vi "(SubVI)DW7912.vi"() -> ()   [LabVIEW 2020]
uses:
  Controls/(Ctrl)DW7912_Wave Seq.ctl
  System Command/Controls/(Ctrl)System Command_Trig GPIO Control.ctl
  <vilib>/Utility/miscctls.llb/LVPointTypeDef.ctl
  Control Data/Controls/(Ctrl)Control Data_Save or Load Control Data_Function.ctl
  Libraries/Haptic IC Class/Haptic IC/Haptic IC.lvclass/Haptic IC.ctl
  I2C/Controls/(Ctrl)I2C_8Bit_Read Array.ctl
  Waveform Editor/Controls/(Ctrl)Waveform Editor_Update Sampling Rate Value.ctl
  a7fdcbe2-e318-4fc3-ac41-e38a3fe8abb3.vi
  Libraries/Haptic IC Class/Haptic IC/Accessors/Write freq ref.vi
  Libraries/Haptic IC Class/Haptic IC/Accessors/Write voltage range ref.vi
  Libraries/Haptic IC Class/Haptic IC/Accessors/Write mode ref.vi
  Variables/(Var)System Variables.vi
  I2C/Instance VIs/(SubVI)I2C_8Bit-8Bit_Read_Single.vi
  I2C/Instance VIs/(SubVI)I2C_8Bit-8Bit_Read_Array.vi
  I2C/Instance VIs/(SubVI)I2C_8Bit-8Bit_Read_Sequential.vi
  I2C/Instance VIs/(SubVI)I2C_8Bit-8Bit_Write_Single.vi
  <vilib>/Comparison/Equal/Equal Functor/Equal Functor.lvclass
  Libraries/Haptic IC Class/Haptic IC/Haptic IC.lvclass
panel:
  in  "Stop":bool
  in  "Read All":bool
  in  "Mode Tab":enum32{"Memory Mode", "Trig Mode"}(tab)
  in  "Mem_Stop":bool
  in  "Mem_Start":bool
  in  "Mem Set_Main Seq Loop":u8(ring) caption="Sequence Loop" items=["X1", "X2", "X3", "X4", "X5", "X6", "X7", "X8", "X9", "X10", "X11", "X12", "X13", "X14", "X15", "Infinite"]
  in  "Mem Set_Gain":u8(ring) caption="MEM Gain" items=["100%", "75%", "50%", "25%"]
  in  "Mem Set_Wave Seq Loop":T1 {"Loop 7" items=["X1", "X2", "X3", "X4", "X5", "X6", "X7", "X8", "X9", "X10", "X11", "X12", "X13", "X14", "X15", "Infinite"]; "Loop 6" items=["X1", "X2", "X3", "X4", "X5", "X6", "X7", "X8", "X9", "X10", "X11", "X12", "X13", "X14", "X15", "Infinite"]; "Loop 5" items=["X1", "X2", "X3", "X4", "X5", "X6", "X7", "X8", "X9", "X10", "X11", "X12", "X13", "X14", "X15", "Infinite"]; "Loop 4" items=["X1", "X2", "X3", "X4", "X5", "X6", "X7", "X8", "X9", "X10", "X11", "X12", "X13", "X14", "X15", "Infinite"]; "Loop 3" items=["X1", "X2", "X3", "X4", "X5", "X6", "X7", "X8", "X9", "X10", "X11", "X12", "X13", "X14", "X15", "Infinite"]; "Loop 2" items=["X1", "X2", "X3", "X4", "X5", "X6", "X7", "X8", "X9", "X10", "X11", "X12", "X13", "X14", "X15", "Infinite"]; "Loop 1" items=["X1", "X2", "X3", "X4", "X5", "X6", "X7", "X8", "X9", "X10", "X11", "X12", "X13", "X14", "X15", "Infinite"]; "Loop 0" items=["X1", "X2", "X3", "X4", "X5", "X6", "X7", "X8", "X9", "X10", "X11", "X12", "X13", "X14", "X15", "Infinite"]}
  in  "Mem Set_Read":bool caption="Wave Sequence"
  in  "Mem Set_Wave Seq":T3 caption="WAVE SEQUENCE" {"Wave Seq. 7"."Seq/Delay" items=["Empty", "1", "2", "3", "4", "5", "6", "7", "8", "9", "10", "11", "12", "13", "14", "15", "16", "17", "18", "19", "20", "21", "22", "23", "24", "25", "26", "27", "28", "29", "30", "31", "32", "33", "34", "35", "36", "37", "38", "39", "40", "41", "42", "43", "44", "45", "46", "47", "48", "49", "50", "51", "52", "53", "54", "55", "56", "57", "58", "59", "60", "61", "62", "63", "64", "65", "66", "67", "68", "69", "70", "71", "72", "73", "74", "75", "76", "77", "78", "79", "80", "81", "82", "83", "84", "85", "86", "87", "88", "89", "90", "91", "92", "93", "94", "95", "96", "97", "98", "99", "100", "101", "102", "103", "104", "105", "106", "107", "108", "109", "110", "111", "112", "113", "114", "115", "116", "117", "118", "119", "120", "121", "122", "123", "124", "125", "126", "127"]; "Wave Seq. 7"."Mode" items=["Wave Seq. 7", "Delay"]; "Wave Seq. 6"."Seq/Delay" items=["Empty", "1", "2", "3", "4", "5", "6", "7", "8", "9", "10", "11", "12", "13", "14", "15", "16", "17", "18", "19", "20", "21", "22", "23", "24", "25", "26", "27", "28", "29", "30", "31", "32", "33", "34", "35", "36", "37", "38", "39", "40", "41", "42", "43", "44", "45", "46", "47", "48", "49", "50", "51", "52", "53", "54", "55", "56", "57", "58", "59", "60", "61", "62", "63", "64", "65", "66", "67", "68", "69", "70", "71", "72", "73", "74", "75", "76", "77", "78", "79", "80", "81", "82", "83", "84", "85", "86", "87", "88", "89", "90", "91", "92", "93", "94", "95", "96", "97", "98", "99", "100", "101", "102", "103", "104", "105", "106", "107", "108", "109", "110", "111", "112", "113", "114", "115", "116", "117", "118", "119", "120", "121", "122", "123", "124", "125", "126", "127"]; "Wave Seq. 6"."Mode" items=["Wave Seq. 6", "Delay"]; "Wave Seq. 5"."Seq/Delay" items=["Empty", "1", "2", "3", "4", "5", "6", "7", "8", "9", "10", "11", "12", "13", "14", "15", "16", "17", "18", "19", "20", "21", "22", "23", "24", "25", "26", "27", "28", "29", "30", "31", "32", "33", "34", "35", "36", "37", "38", "39", "40", "41", "42", "43", "44", "45", "46", "47", "48", "49", "50", "51", "52", "53", "54", "55", "56", "57", "58", "59", "60", "61", "62", "63", "64", "65", "66", "67", "68", "69", "70", "71", "72", "73", "74", "75", "76", "77", "78", "79", "80", "81", "82", "83", "84", "85", "86", "87", "88", "89", "90", "91", "92", "93", "94", "95", "96", "97", "98", "99", "100", "101", "102", "103", "104", "105", "106", "107", "108", "109", "110", "111", "112", "113", "114", "115", "116", "117", "118", "119", "120", "121", "122", "123", "124", "125", "126", "127"]; "Wave Seq. 5"."Mode" items=["Wave Seq. 5", "Delay"]; "Wave Seq. 4"."Seq/Delay" items=["Empty", "1", "2", "3", "4", "5", "6", "7", "8", "9", "10", "11", "12", "13", "14", "15", "16", "17", "18", "19", "20", "21", "22", "23", "24", "25", "26", "27", "28", "29", "30", "31", "32", "33", "34", "35", "36", "37", "38", "39", "40", "41", "42", "43", "44", "45", "46", "47", "48", "49", "50", "51", "52", "53", "54", "55", "56", "57", "58", "59", "60", "61", "62", "63", "64", "65", "66", "67", "68", "69", "70", "71", "72", "73", "74", "75", "76", "77", "78", "79", "80", "81", "82", "83", "84", "85", "86", "87", "88", "89", "90", "91", "92", "93", "94", "95", "96", "97", "98", "99", "100", "101", "102", "103", "104", "105", "106", "107", "108", "109", "110", "111", "112", "113", "114", "115", "116", "117", "118", "119", "120", "121", "122", "123", "124", "125", "126", "127"]; "Wave Seq. 4"."Mode" items=["Wave Seq. 4", "Delay"]; "Wave Seq. 3"."Seq/Delay" items=["Empty", "1", "2", "3", "4", "5", "6", "7", "8", "9", "10", "11", "12", "13", "14", "15", "16", "17", "18", "19", "20", "21", "22", "23", "24", "25", "26", "27", "28", "29", "30", "31", "32", "33", "34", "35", "36", "37", "38", "39", "40", "41", "42", "43", "44", "45", "46", "47", "48", "49", "50", "51", "52", "53", "54", "55", "56", "57", "58", "59", "60", "61", "62", "63", "64", "65", "66", "67", "68", "69", "70", "71", "72", "73", "74", "75", "76", "77", "78", "79", "80", "81", "82", "83", "84", "85", "86", "87", "88", "89", "90", "91", "92", "93", "94", "95", "96", "97", "98", "99", "100", "101", "102", "103", "104", "105", "106", "107", "108", "109", "110", "111", "112", "113", "114", "115", "116", "117", "118", "119", "120", "121", "122", "123", "124", "125", "126", "127"]; "Wave Seq. 3"."Mode" items=["Wave Seq. 3", "Delay"]; "Wave Seq. 2"."Seq/Delay" items=["Empty", "1", "2", "3", "4", "5", "6", "7", "8", "9", "10", "11", "12", "13", "14", "15", "16", "17", "18", "19", "20", "21", "22", "23", "24", "25", "26", "27", "28", "29", "30", "31", "32", "33", "34", "35", "36", "37", "38", "39", "40", "41", "42", "43", "44", "45", "46", "47", "48", "49", "50", "51", "52", "53", "54", "55", "56", "57", "58", "59", "60", "61", "62", "63", "64", "65", "66", "67", "68", "69", "70", "71", "72", "73", "74", "75", "76", "77", "78", "79", "80", "81", "82", "83", "84", "85", "86", "87", "88", "89", "90", "91", "92", "93", "94", "95", "96", "97", "98", "99", "100", "101", "102", "103", "104", "105", "106", "107", "108", "109", "110", "111", "112", "113", "114", "115", "116", "117", "118", "119", "120", "121", "122", "123", "124", "125", "126", "127"]; "Wave Seq. 2"."Mode" items=["Wave Seq. 2", "Delay"]; "Wave Seq. 1"."Seq/Delay" items=["Empty", "1", "2", "3", "4", "5", "6", "7", "8", "9", "10", "11", "12", "13", "14", "15", "16", "17", "18", "19", "20", "21", "22", "23", "24", "25", "26", "27", "28", "29", "30", "31", "32", "33", "34", "35", "36", "37", "38", "39", "40", "41", "42", "43", "44", "45", "46", "47", "48", "49", "50", "51", "52", "53", "54", "55", "56", "57", "58", "59", "60", "61", "62", "63", "64", "65", "66", "67", "68", "69", "70", "71", "72", "73", "74", "75", "76", "77", "78", "79", "80", "81", "82", "83", "84", "85", "86", "87", "88", "89", "90", "91", "92", "93", "94", "95", "96", "97", "98", "99", "100", "101", "102", "103", "104", "105", "106", "107", "108", "109", "110", "111", "112", "113", "114", "115", "116", "117", "118", "119", "120", "121", "122", "123", "124", "125", "126", "127"]; "Wave Seq. 1"."Mode" items=["Wave Seq. 1", "Delay"]; "Wave Seq. 0"."Seq/Delay" items=["Empty", "1", "2", "3", "4", "5", "6", "7", "8", "9", "10", "11", "12", "13", "14", "15", "16", "17", "18", "19", "20", "21", "22", "23", "24", "25", "26", "27", "28", "29", "30", "31", "32", "33", "34", "35", "36", "37", "38", "39", "40", "41", "42", "43", "44", "45", "46", "47", "48", "49", "50", "51", "52", "53", "54", "55", "56", "57", "58", "59", "60", "61", "62", "63", "64", "65", "66", "67", "68", "69", "70", "71", "72", "73", "74", "75", "76", "77", "78", "79", "80", "81", "82", "83", "84", "85", "86", "87", "88", "89", "90", "91", "92", "93", "94", "95", "96", "97", "98", "99", "100", "101", "102", "103", "104", "105", "106", "107", "108", "109", "110", "111", "112", "113", "114", "115", "116", "117", "118", "119", "120", "121", "122", "123", "124", "125", "126", "127"]; "Wave Seq. 0"."Mode" items=["Wave Seq. 0", "Delay"]}
  out "Trig_Gen_Pict":picture
  in  "Trig_Read":bool caption="Trig/Interrupt Mode Set"
  in  "Trig_Gen_Set":bool
  in  "Trig_Mode":bool
  in  "Trig_F Wave":u8(ring) caption="TRIG F Wave" items=["Empty", "1", "2", "3", "4", "5", "6", "7", "8", "9", "10", "11", "12", "13", "14", "15", "16", "17", "18", "19", "20", "21", "22", "23", "24", "25", "26", "27", "28", "29", "30", "31", "32", "33", "34", "35", "36", "37", "38", "39", "40", "41", "42", "43", "44", "45", "46", "47", "48", "49", "50", "51", "52", "53", "54", "55", "56", "57", "58", "59", "60", "61", "62", "63", "64", "65", "66", "67", "68", "69", "70", "71", "72", "73", "74", "75", "76", "77", "78", "79", "80", "81", "82", "83", "84", "85", "86", "87", "88", "89", "90", "91", "92", "93", "94", "95", "96", "97", "98", "99", "100", "101", "102", "103", "104", "105", "106", "107", "108", "109", "110", "111", "112", "113", "114", "115", "116", "117", "118", "119", "120", "121", "122", "123", "124", "125", "126", "127"]
  in  "Trig_R Wave":u8(ring) caption="TRIG R Wave" items=["Empty", "1", "2", "3", "4", "5", "6", "7", "8", "9", "10", "11", "12", "13", "14", "15", "16", "17", "18", "19", "20", "21", "22", "23", "24", "25", "26", "27", "28", "29", "30", "31", "32", "33", "34", "35", "36", "37", "38", "39", "40", "41", "42", "43", "44", "45", "46", "47", "48", "49", "50", "51", "52", "53", "54", "55", "56", "57", "58", "59", "60", "61", "62", "63", "64", "65", "66", "67", "68", "69", "70", "71", "72", "73", "74", "75", "76", "77", "78", "79", "80", "81", "82", "83", "84", "85", "86", "87", "88", "89", "90", "91", "92", "93", "94", "95", "96", "97", "98", "99", "100", "101", "102", "103", "104", "105", "106", "107", "108", "109", "110", "111", "112", "113", "114", "115", "116", "117", "118", "119", "120", "121", "122", "123", "124", "125", "126", "127"]
  in  "Trig_Gen_Setting":T4={"1st Trig"={"Trigger"=TRUE, "Low"=0, "High"=100}, "2nd Trig"={"Trigger"=TRUE, "Low"=0, "High"=100}, "3rd Trig"={"Trigger"=FALSE, "Low"=0, "High"=1}, "4th Trig"={"Trigger"=FALSE, "Low"=0, "High"=1}} {"4th Trig"."High" min=1 max=8000; "4th Trig"."Low" max=7999; "3rd Trig"."High" min=1 max=8000; "3rd Trig"."Low" max=7999; "2nd Trig"."High" min=1 max=8000; "2nd Trig"."Low" max=7999; "1st Trig"."High" min=1 max=8000; "1st Trig"."Low" max=7999}
  in  "Common Tab":enum32{"Common"}(tab)
  in  "Com_Status_Read":bool
  in  "Com_Read":bool caption="Common"
  in  "Com_Bst_VD Clamp":u8(ring) caption="VD Clamp" items=["0.00V", "0.04V", "0.08V", "0.12V", "0.16V", "0.20V", "0.24V", "0.28V", "0.32V", "0.36V", "0.40V", "0.44V", "0.48V", "0.52V", "0.56V", "0.60V", "0.64V", "0.68V", "0.72V", "0.76V", "0.80V", "0.84V", "0.88V", "0.92V", "0.96V", "1.00V", "1.04V", "1.08V", "1.12V", "1.16V", "1.20V", "1.24V", "1.28V", "1.32V", "1.36V", "1.40V", "1.44V", "1.48V", "1.52V", "1.56V", "1.60V", "1.64V", "1.68V", "1.72V", "1.76V", "1.80V", "1.84V", "1.88V", "1.92V", "1.96V", "2.00V", "2.04V", "2.08V", "2.12V", "2.16V", "2.20V", "2.24V", "2.28V", "2.32V", "2.36V", "2.40V", "2.44V", "2.48V", "2.52V", "2.56V", "2.60V", "2.64V", "2.68V", "2.72V", "2.76V", "2.80V", "2.84V", "2.88V", "2.92V", "2.96V", "3.00V", "3.04V", "3.08V", "3.12V", "3.16V", "3.20V", "3.24V", "3.28V", "3.32V", "3.36V", "3.40V", "3.44V", "3.48V", "3.52V", "3.56V", "3.60V", "3.64V", "3.68V", "3.72V", "3.76V", "3.80V", "3.84V", "3.88V", "3.92V", "3.96V", "4.00V", "4.04V", "4.08V", "4.12V", "4.16V", "4.20V", "4.24V", "4.28V", "4.32V", "4.36V", "4.40V", "4.44V", "4.48V", "4.52V", "4.56V", "4.60V", "4.64V", "4.68V", "4.72V", "4.76V", "4.80V", "4.84V", "4.88V", "4.92V", "4.96V", "5.00V", "5.04V", "5.08V", "5.12V", "5.16V", "5.20V", "5.24V", "5.28V", "5.32V", "5.36V", "5.40V", "5.44V", "5.48V", "5.52V", "5.56V", "5.60V", "5.64V", "5.68V", "5.72V", "5.76V", "5.80V", "5.84V", "5.88V", "5.92V", "5.96V", "6.00V", "6.04V", "6.08V", "6.12V", "6.16V", "6.20V", "6.24V", "6.28V", "6.32V", "6.36V", "6.40V", "6.44V", "6.48V", "6.52V", "6.56V", "6.60V", "6.64V", "6.68V", "6.72V", "6.76V", "6.80V", "6.84V", "6.88V", "6.92V", "6.96V", "7.00V", "7.04V", "7.08V", "7.12V", "7.16V", "7.20V", "7.24V", "7.28V", "7.32V", "7.36V", "7.40V", "7.44V", "7.48V", "7.52V", "7.56V", "7.60V", "7.64V", "7.68V", "7.72V", "7.76V", "7.80V", "7.84V", "7.88V", "7.92V", "7.96V", "8.00V", "8.04V", "8.08V", "8.12V", "8.16V", "8.20V", "8.24V", "8.28V", "8.32V", "8.36V", "8.40V", "8.44V", "8.48V", "8.52V", "8.56V", "8.60V", "8.64V", "8.68V", "8.72V", "8.76V", "8.80V", "8.84V", "8.88V", "8.92V", "8.96V", "9.00V", "9.04V", "9.08V", "9.12V", "9.16V", "9.20V", "9.24V", "9.28V", "9.32V", "9.36V", "9.40V", "9.44V", "9.48V", "9.52V", "9.56V", "9.60V", "9.64V", "9.68V", "9.72V", "9.76V", "9.80V", "9.84V", "9.88V", "9.92V", "9.96V", "10.00V", "10.04V", "10.08V", "10.12V", "10.16V", "10.20V"]
  in  "Com_Bst_Wait":u8(ring) caption="Wait Time" items=["0us", "166us", "332us", "498us", "664us", "830us", "996us", "1162us", "1328us", "1494us", "1660us", "1826us", "1992us", "2158us", "2324us", "2490us"]
  in  "Com_Bst_VD Clamp Reg":u8(ring) caption="VD Clamp Reg" items=["Header", "VD Clamp"]
  in  "Com_Mode":enum16{"RTP Mode", "MEM Mode"}(ring) caption="Mode"
  in  "Com_Bst_Mode":u8(ring)=4 caption="Mode" items=["Bypass"=2, "Lump"=4, "Adapt"=8]
  in  "Com_Bst_Offset":u8(ring) caption="BST Offset" items=["0.00V", "0.08V", "0.16V", "0.24V", "0.32V", "0.40V", "0.48V", "0.56V", "0.64V", "0.72V", "0.80V", "0.88V", "0.96V", "1.04V", "1.12V", "1.20V", "1.28V", "1.36V", "1.44V", "1.52V", "1.60V", "1.68V", "1.76V", "1.84V", "1.92V", "2.00V", "2.08V", "2.16V", "2.24V", "2.32V", "2.40V", "2.48V"]
  in  "Com_Bst_Limit":u8(ring) caption="BST Limit" items=["3.0A", "2.5A", "2.0A", "1.5A", "3.5A"]
  in  "Com_PWM Freq":u8(ring)=1 caption="PWM Freq." items=["24kHz", "48kHz", "96kHz", "12kHz"]
  out "Com_Status_Result":string caption="Result :"
  # "WAVE SEQ CTRL"
  # "Wave Seq."
  # "Mem No."
  # "Loop"
  # "TRIG CTRL"
  # "TRIG1/2 WAVE CTRL"
  # "TRIGGER GENERATOR"
  # "Trigger"
  # "R (ms)"
  # "F (ms)"
  # "STATUS READ"
  # "MODE"
  # "PWM FREQ / ETC"
  # "BOOST MODE"
  # "VD CLAMP"
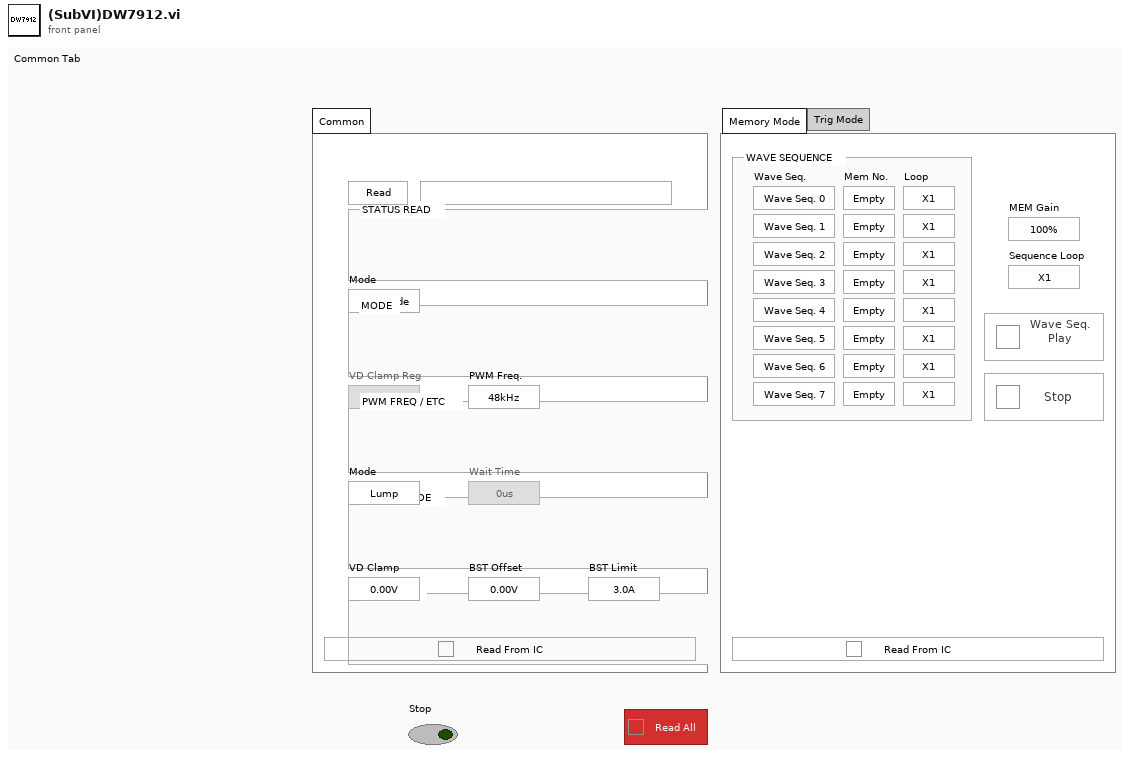
[diagram p1: front panel]
types:
  T1 = cluster{"Loop 0":u8, "Loop 1":u8, "Loop 2":u8, "Loop 3":u8, "Loop 4":u8, "Loop 5":u8, "Loop 6":u8, "Loop 7":u8}
  T2 = typedef "(Ctrl)DW7912_Wave Seq.ctl" = cluster{"Mode":u8, "Seq/Delay":u8}
  T3 = cluster{"Wave Seq. 0":T2, "Wave Seq. 1":T2, "Wave Seq. 2":T2, "Wave Seq. 3":T2, "Wave Seq. 4":T2, "Wave Seq. 5":T2, "Wave Seq. 6":T2, "Wave Seq. 7":T2}
  T4 = typedef "(Ctrl)System Command_Trig GPIO Control.ctl" = cluster{"1st Trig":cluster{"Trigger":bool, "Low":u16, "High":u16}, "2nd Trig":cluster{"Trigger":bool, "Low":u16, "High":u16}, "3rd Trig":cluster{"Trigger":bool, "Low":u16, "High":u16}, "4th Trig":cluster{"Trigger":bool, "Low":u16, "High":u16}}
  T5 = enum8{"Enabled", "Disabled", "Disabled and Grayed Out"}
  T6 = typedef "(Ctrl)Control Data_Save or Load Control Data_Function.ctl" = enum16{"Save", "Load"}
  T7 = typedef "LVPointTypeDef.ctl" = cluster{"Horizontal":i16, "Vertical":i16}
  T8 = typedef "(Ctrl)I2C_8Bit_Read Array.ctl" = cluster{"Address":u8, "Delay(ms)":i32}
  T9 = typedef "(Ctrl)Waveform Editor_Update Sampling Rate Value.ctl" = enum16{"Init", "Update"}
  T10 = cluster{"[0]":cluster{u8, u8}, "[1]":cluster{u8, u8}, "[2]":cluster{u8, u8}, "[3]":cluster{u8, u8}, "[4]":cluster{u8, u8}, "[5]":cluster{u8, u8}, "[6]":cluster{u8, u8}, "[7]":cluster{u8, u8}}
  T11 = cluster{"[0]":u8, "[1]":u8, "[2]":u8, "[3]":u8, "[4]":u8, "[5]":u8, "[6]":u8, "[7]":u8}
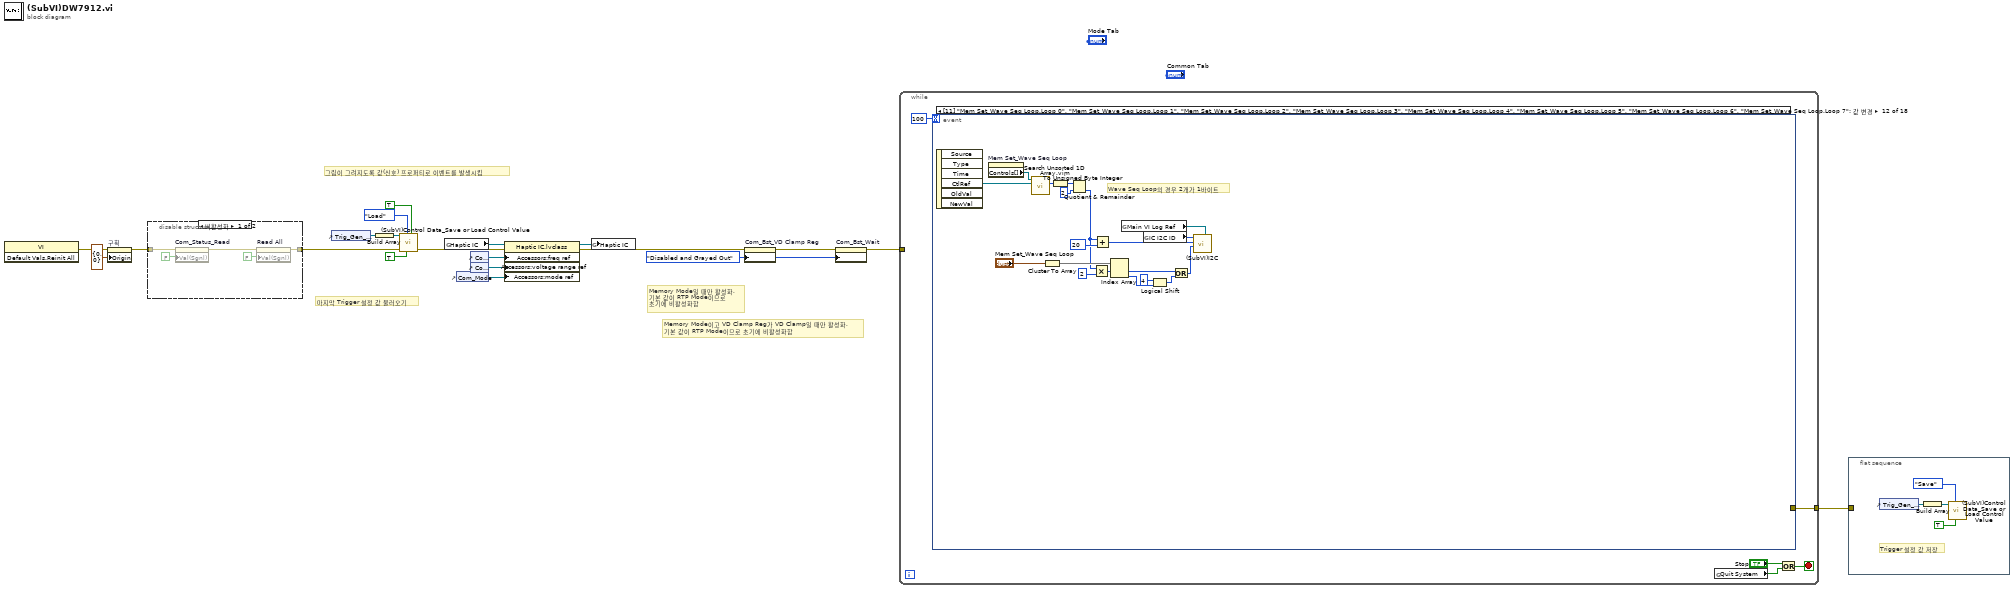
[diagram p0: block diagram]
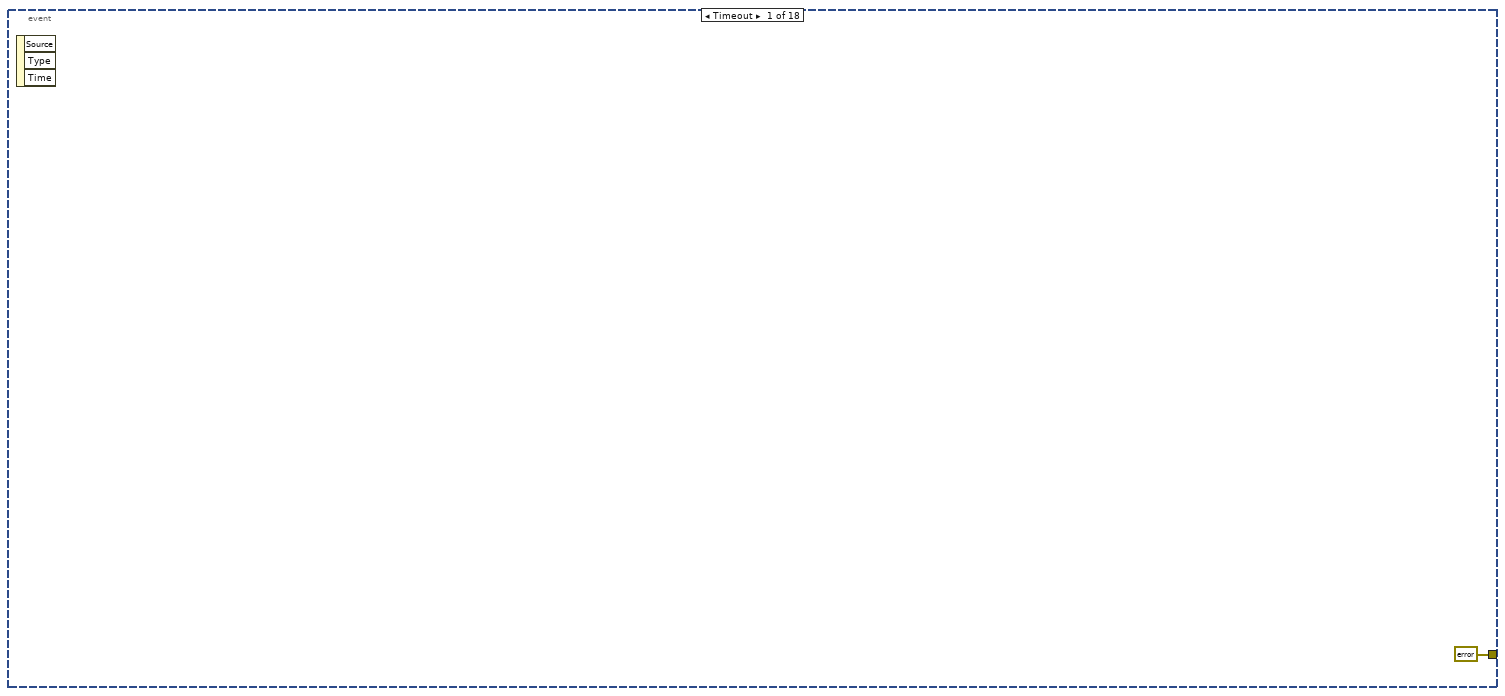
[diagram p3: hidden frame]
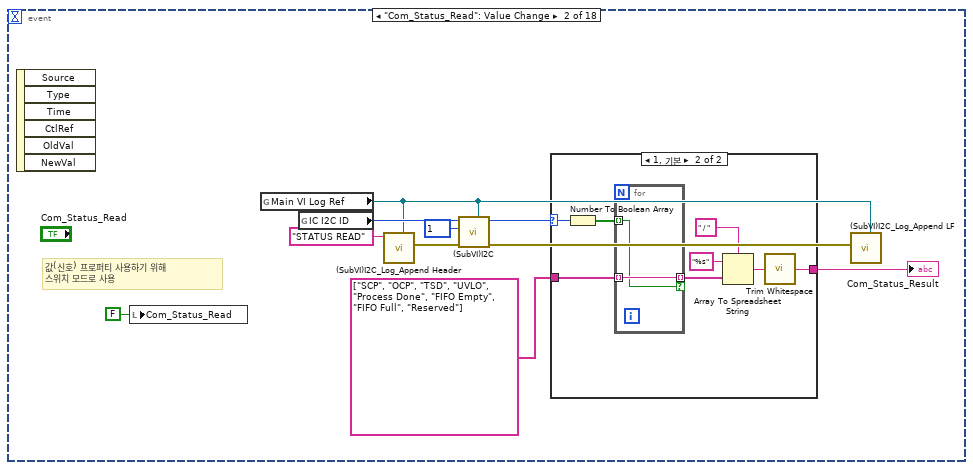
[diagram p4: hidden frame]
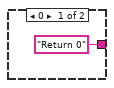
[diagram p5: hidden frame]
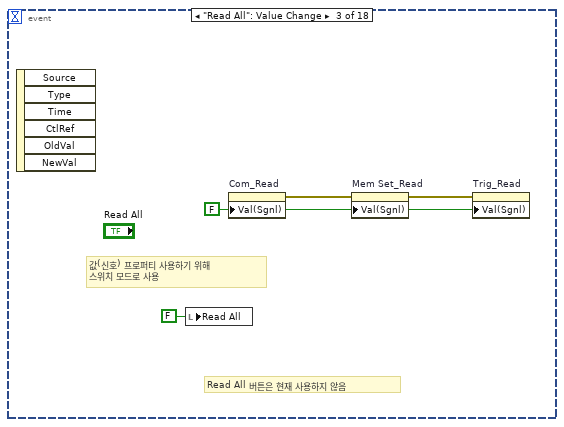
[diagram p6: hidden frame]
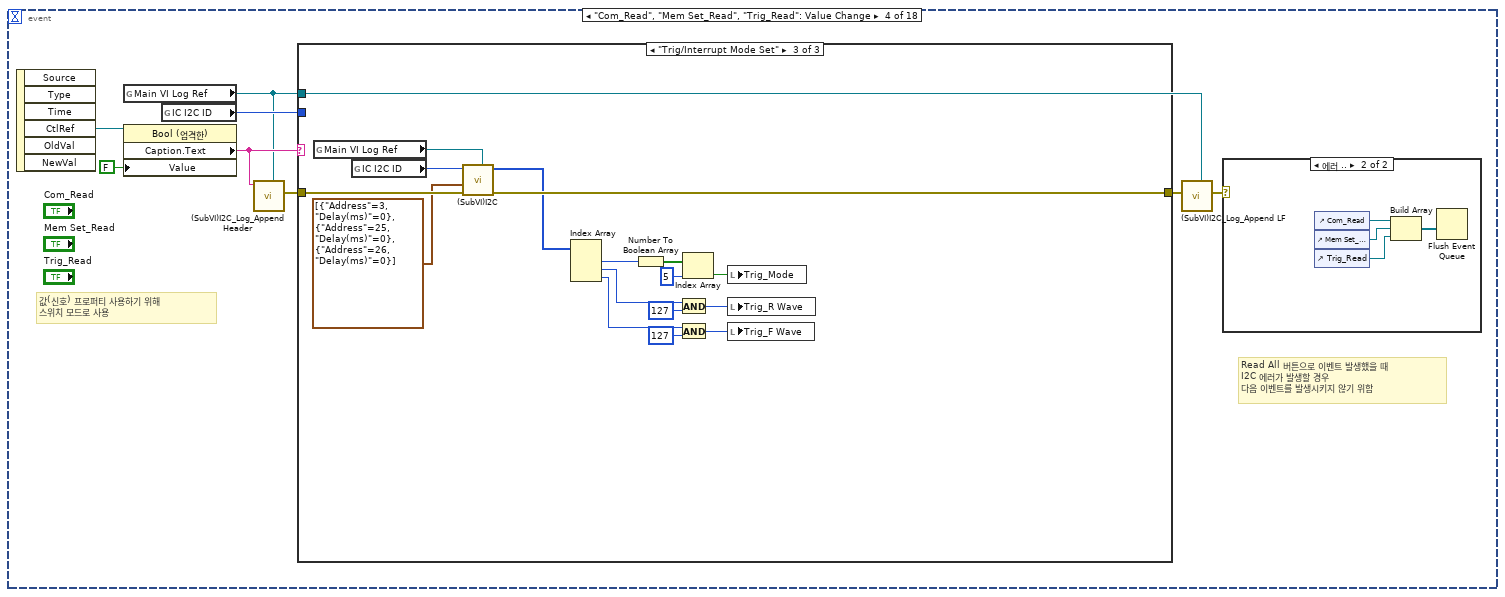
[diagram p7: hidden frame]
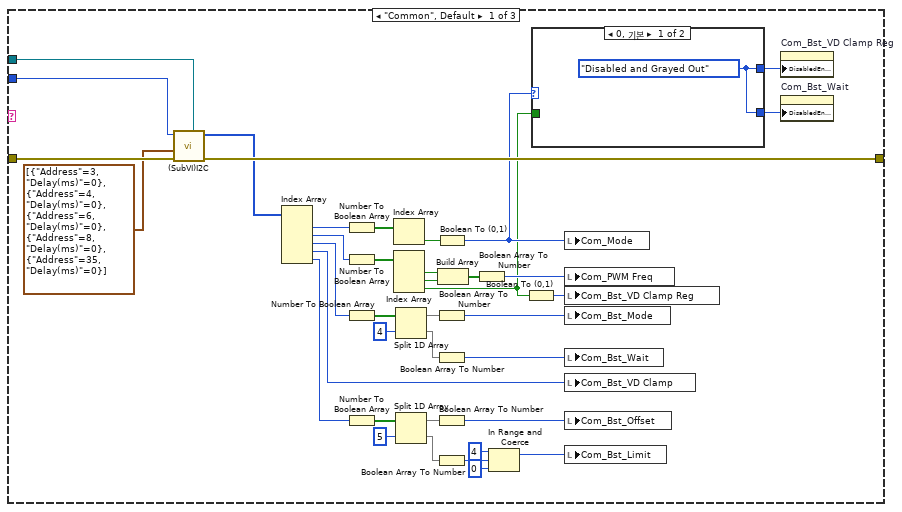
[diagram p8: hidden frame]
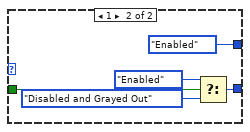
[diagram p9: hidden frame]
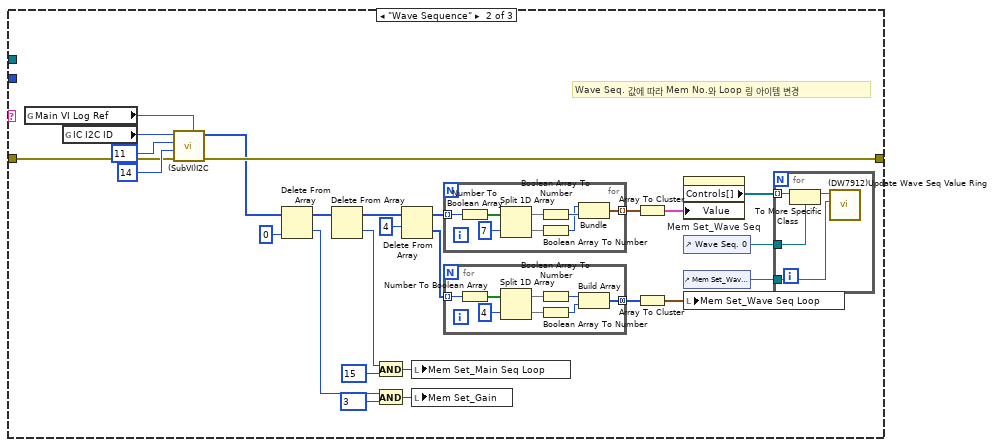
[diagram p10: hidden frame]
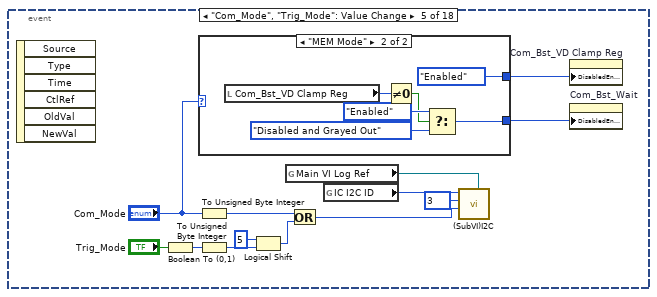
[diagram p12: hidden frame]
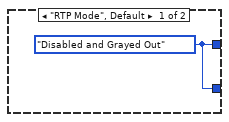
[diagram p13: hidden frame]
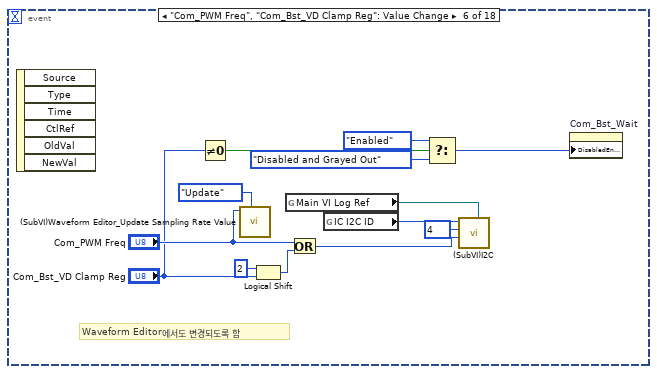
[diagram p14: hidden frame]
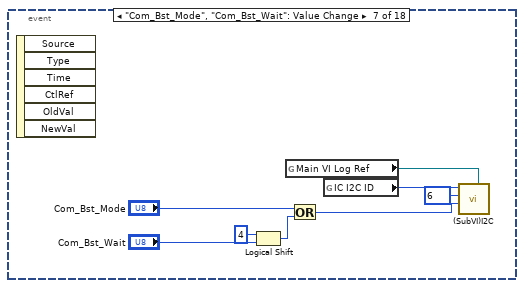
[diagram p15: hidden frame]
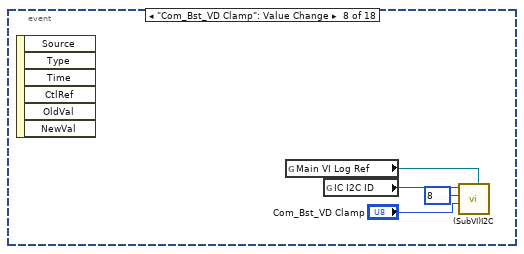
[diagram p16: hidden frame]
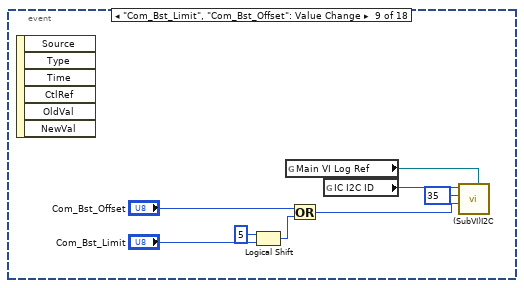
[diagram p17: hidden frame]
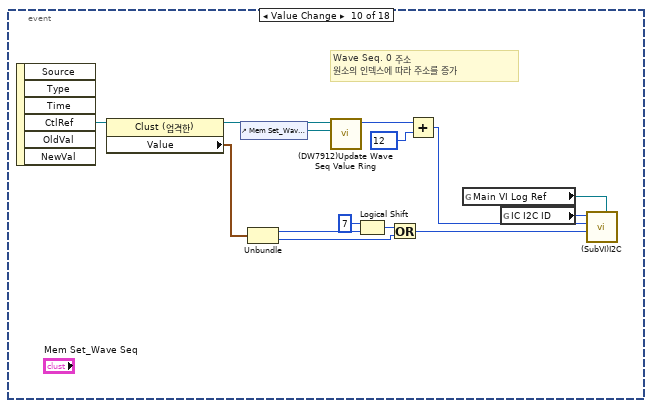
[diagram p18: hidden frame]
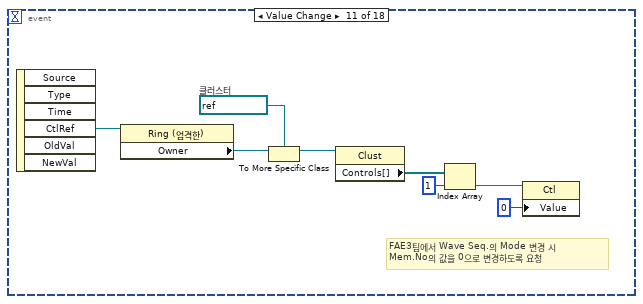
[diagram p19: hidden frame]
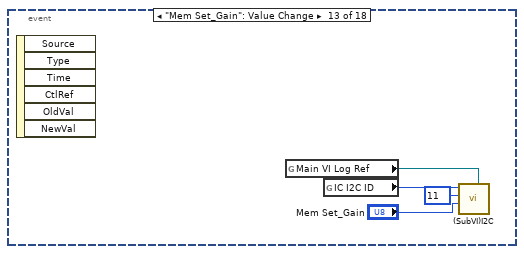
[diagram p20: hidden frame]
diagram:
  w2 = T5."Disabled and Grayed Out" ("비활성화")
  # "그림이 그려지도록 값(신호) 프로퍼티로 이벤트를 발생시킴"
  # "Memory Mode이고 VD Clamp Reg가 VD Clamp일 때만 활성화,\n기본 값이 RTP Mode이므로 초기에 비활성화함"
  # "Memory Mode일 때만 활성화,\n기본 값이 RTP Mode이므로\n초기에 비활성화함"
  # "마지막 Trigger 설정 값 불러오기"
  n1 = invoke class="VI" method="Default Vals.Reinit All"() -> (error out=w20:errorcluster)  [unwired: 3 in, 2 out]
  n2 = property on="구획" class="Pane"(error in=w20, "Origin"=T7 {"Horizontal"=0, "Vertical"=0} ("원점")) -> (error out=w12:errorcluster)  [unwired: 1 in, 1 out]
  n3 = disable-structure shown="비활성화" {
    disable-tunnel: [w24 w26] -> w14
    disable-tunnel: w12 -> [w23 w26]
    frame Disabled {
      n4 = property on="Com_Status_Read" class="Bool (엄격한)"(error in=w23, "Val(Sgnl)"=FALSE ("값(신호)")) -> (error out=w22:errorcluster)  [unwired: 1 in, 1 out]
      n5 = property on="Read All" class="Bool (엄격한)"(error in=w22, "Val(Sgnl)"=FALSE ("값(신호)")) -> (error out=w24:errorcluster)  [unwired: 1 in, 1 out]
    }
    frame Enabled {
    }
  }
  n6 = control-ref of="Trig_Gen_Setting"() -> (w15:refnum<vi>)
  n7 = Build Array(w15) -> (w16:refnum<vi>[])
  n8 = call "(SubVI)Control Data_Save or Load Control Value.vi"("Val(Sgnl)"=TRUE, "Common? (f)"=TRUE, "Function"=(Ctrl)Control_Data_Save_or_Load_Control_Data_Function."Load", "error in (no error)"=w14, "Control Ref"=w16) -> ("error out"=w10:errorcluster)  [unwired: 6 in]
  n9 = global read "(Var)System Variables.vi" "Haptic IC"() -> (w11:refnum<class "Haptic IC.lvclass">)
  n10 = control-ref of="Com_Mode"() -> (w7:refnum<vi>)
  n11 = control-ref of="Com_PWM Freq"() -> (w9:refnum<vi>)
  n12 = control-ref of="Com_Bst_VD Clamp"() -> (w8:refnum<vi>)
  n13 = property class="Haptic IC.lvclass"(reference=w11, error in=w10, "Accessors:freq ref"=w9, "Accessors:voltage range ref"=w8, "Accessors:mode ref"=w7) -> (reference out=w6:refnum<class "Haptic IC.lvclass">, error out=w4:errorcluster)
  n14 = global write "(Var)System Variables.vi" "Haptic IC"(w6) -> ()
  n15 = property on="Com_Bst_VD Clamp Reg" class="Ring (엄격한)"(error in=w4, "DisabledEnum"=w2) -> (error out=w3:errorcluster)  [unwired: 1 in, 1 out]
  n16 = property on="Com_Bst_Wait" class="Ring (엄격한)"(error in=w3, "DisabledEnum"=w2) -> (error out=w1:errorcluster)  [unwired: 1 in, 1 out]
  n17 = while {
    tunnel: [w29] -> w18
    tunnel: w1 -> [_]
    stop <- w28 stop-if-true
    n18 = event shown="[11] \"Mem Set_Wave Seq Loop.Loop 0\", \"Mem Set_Wave Seq Loop.Loop 1\", \"Mem Set_Wave Seq Loop.Loop 2\", \"Mem Set_Wave Seq Loop.Loop 3\", \"Mem Set_Wave Seq Loop.Loop 4\", \"Mem Set_Wave Seq Loop.Loop 5\", \"Mem Set_Wave Seq Loop.Loop 6\", \"Mem Set_Wave Seq Loop.Loop 7\": 값 변경" {
      selector: _ -> [_ _ _ _ _ _ _ _ _ _ _ _ _ _ _ _ _ _]
      dyn-events: _ -> [_ _ _ _ _ _ _ _ _ _ _ _ _ _ _ _ _ _]
      timeout: 100 -> [_ _ _ _ _ _ _ _ _ _ _ _ _ _ _ _ _ _]
      tunnel: [errorcluster {"status"=FALSE, "code"=0, "source"=""} ("에러 상수") _ _ _ _ _ _ _ _ _ _ _ _ _ _ _ _ _] -> w29
      event Timeout {
        n19 = event-data() -> ()  [unwired: 1 in, 3 out]
      }
      event "Com_Status_Read": Value Change {
        # "값(신호) 프로퍼티 사용하기 위해\n스위치 모드로 사용"
        n20 = event-data() -> ()  [unwired: 1 in, 6 out]
        n21 = local write "Com_Status_Read"(FALSE ("Com_Status_Read")) -> ()
        n22 = global read "(Var)System Variables.vi" "Main VI Log Ref"() -> (w34:refnum<vi>)
        n23 = global read "(Var)System Variables.vi" "IC I2C ID"() -> (w42:u8)
        n24 = call "(SubVI)I2C_Log_Append Header.vi"("Log Ref"=w34, "Header"="STATUS READ") -> ("error out"=w38:errorcluster)  [unwired: 9 in]
        n25 = call-poly "(SubVI)I2C.vi"("Log Ref"=w34, "error in (no error)"=w38, "Address"=u8 1, "ID"=w42) -> ("error out"=w35:errorcluster, "Read Data"=w39:u8)  [unwired: 5 in, 1 out]
        n26 = case shown="1, 기본" w39 {
          selector: w39 -> [_ w51]
          tunnel: string[] ["SCP", "OCP", "TSD", "UVLO", "Process Done", "FIFO Empty", "FIFO Full", "Reserved"] -> [_ w49]
          tunnel: ["Return 0" ("trimmed string") w44] -> w36
          frame 0 {
          }
          frame 1, Default {
            n27 = Number To Boolean Array(number=w51) -> (Boolean array=w50:bool[])
            n28 = for {
              tunnel: w50 -> [w52] mode=indexing
              tunnel: w49 -> [w53] mode=indexing
              tunnel: [w53] -> w48 mode=indexing if=w52
            }
            n29 = Array To Spreadsheet String(delimiter (Tab)=" / " ("구분 문자 (탭)"), array=w48, 3:"%s" ("포맷 문자열")) -> (spreadsheet string=w45:string)
            n30 = call <vilib>:"Trim Whitespace.vi"("string"=w45) -> ("trimmed string"=w44:string)  [unwired: 1 in]
          }
        }
        "Com_Status_Result" <- w36
        n31 = call "(SubVI)I2C_Log_Append LF.vi"("Log Ref"=w34, "error in (no error)"=w35) -> ()  [unwired: 9 in, 1 out]
      }
      event "Read All": Value Change {
        w55 = FALSE ("값(신호)")
        # "Read All 버튼은 현재 사용하지 않음"
        # "값(신호) 프로퍼티 사용하기 위해\n스위치 모드로 사용"
        n32 = event-data() -> ()  [unwired: 1 in, 6 out]
        n33 = local write "Read All"(FALSE ("Read All")) -> ()
        n34 = property on="Com_Read" class="Bool (엄격한)"("Val(Sgnl)"=w55) -> (error out=w57:errorcluster)  [unwired: 2 in, 1 out]
        n35 = property on="Mem Set_Read" class="Bool (엄격한)"(error in=w57, "Val(Sgnl)"=w55) -> (error out=w56:errorcluster)  [unwired: 1 in, 1 out]
        n36 = property on="Trig_Read" class="Bool (엄격한)"(error in=w56, "Val(Sgnl)"=w55) -> ()  [unwired: 1 in, 2 out]
      }
      event "Com_Read", "Mem Set_Read", "Trig_Read": Value Change {
        # "Read All 버튼으로 이벤트 발생했을 때\nI2C 에러가 발생할 경우 \n다음 이벤트를 발생시키지 않기 위함"
        # "값(신호) 프로퍼티 사용하기 위해\n스위치 모드로 사용"
        n37 = event-data() -> ("CtlRef"=w65:refnum<vi>)  [unwired: 1 in, 5 out]
        n38 = global read "(Var)System Variables.vi" "Main VI Log Ref"() -> (w58:refnum<vi>)
        n39 = property class="Bool (엄격한)"(reference=w65, "Value"=FALSE ("값")) -> ("Caption.Text"=w60:string)  [unwired: 1 in, 2 out]
        n40 = global read "(Var)System Variables.vi" "IC I2C ID"() -> (w62:u8)
        n41 = call "(SubVI)I2C_Log_Append Header.vi"("Log Ref"=w58, "Header"=w60) -> ("error out"=w61:errorcluster)  [unwired: 9 in]
        n42 = case shown="\"Trig/Interrupt Mode Set\"" w60 {
          tunnel: [w102 w133 w168] -> w63
          tunnel: w58 -> [w74 _ _]
          tunnel: w62 -> [w73 _ _]
          tunnel: w61 -> [w103 w110 w171]
          frame "Common", Default {
            n43 = call-poly "(SubVI)I2C.vi"("Log Ref"=w74, "error in (no error)"=w103, "Address to Read"=T8[] [{"Address"=3, "Delay(ms)"=0}, {"Address"=4, "Delay(ms)"=0}, {"Address"=6, "Delay(ms)"=0}, {"Address"=8, "Delay(ms)"=0}, {"Address"=35, "Delay(ms)"=0}], "ID"=w73) -> ("error out"=w102:errorcluster, "Read Data"=w100:u8[])  [unwired: 5 in, 1 out]
            n44 = Index Array(array=w100) -> (element #1=w99:u8, element #2=w95:u8, element #3=w94:u8, element #4=w89:u8, element #5=w86:u8)  [unwired: 5 in]
            n45 = Number To Boolean Array(number=w99) -> (Boolean array=w98:bool[])
            n46 = Number To Boolean Array(number=w95) -> (Boolean array=w96:bool[])
            n47 = Number To Boolean Array(number=w94) -> (Boolean array=w93:bool[])
            n48 = Number To Boolean Array(number=w86) -> (Boolean array=w87:bool[])
            n49 = Index Array(array=w98) -> (element=w97:bool)  [unwired: 1 in]
            n50 = Index Array(array=w96) -> (element #1=w78:bool, element #2=w77:bool, element #3=w69:bool)  [unwired: 3 in]
            n51 = Split 1D Array(array=w93, index=4 ("인덱스")) -> (first subarray=w68:bool[], second subarray=w91:bool[])
            n52 = Split 1D Array(array=w87, index=5 ("인덱스")) -> (first subarray=w85:bool[], second subarray=w83:bool[])
            n53 = Boolean To (0,1)(Boolean=w97) -> (0, 1=w70:i16)
            n54 = Boolean Array To Number(Boolean array=w68) -> (number=w67:u32)
            n55 = Boolean Array To Number ("불리언 배열을 숫자로")(Boolean array=w91) -> (number=w90:u8)
            n56 = Boolean Array To Number ("불리언 배열을 숫자로")(Boolean array=w85) -> (number=w84:u8)
            n57 = Boolean Array To Number ("불리언 배열을 숫자로")(Boolean array=w83) -> (number=w82:u8)
            n58 = Build Array(w78, w77) -> (w76:bool[])
            n59 = Boolean Array To Number ("불리언 배열을 숫자로")(Boolean array=w76) -> (number=w75:u8)
            n60 = In Range and Coerce(upper limit=u8 4 ("상위 리미트"), x=w82, lower limit=u8 0 ("하위 리미트")) -> (coerced(x)=w79:u8)  [unwired: 1 out]
            n61 = Boolean To (0,1)(Boolean=w69) -> (0, 1=w66:i16)
            n62 = case shown="0, 기본" w70 {
              tunnel: [w104 T5."Enabled" ("비활성화")] -> w72
              tunnel: [w104 w106] -> w71
              tunnel: w69 -> [_ w105]
              frame 0, Default {
                w104 = T5."Disabled and Grayed Out" ("비활성화")
              }
              frame 1 {
                n63 = Select(t=T5."Enabled" ("비활성화"), s=w105, f=T5."Disabled and Grayed Out") -> (s? t:f=w106:T5)
              }
            }
            n64 = local write "Com_Mode"(w70) -> ()
            n65 = local write "Com_PWM Freq"(w75) -> ()
            n66 = local write "Com_Bst_VD Clamp Reg"(w66) -> ()
            n67 = local write "Com_Bst_Mode"(w67) -> ()
            n68 = local write "Com_Bst_Wait"(w90) -> ()
            n69 = local write "Com_Bst_VD Clamp"(w89) -> ()
            n70 = local write "Com_Bst_Offset"(w84) -> ()
            n71 = local write "Com_Bst_Limit"(w79) -> ()
            n72 = property on="Com_Bst_VD Clamp Reg" class="Ring (엄격한)"("DisabledEnum"=w72) -> ()  [unwired: 2 in, 2 out]
            n73 = property on="Com_Bst_Wait" class="Ring (엄격한)"("DisabledEnum"=w71) -> ()  [unwired: 2 in, 2 out]
          }
          frame "Wave Sequence" {
            # "Wave Seq. 값에 따라 Mem No.와 Loop 링 아이템 변경"
            n74 = global read "(Var)System Variables.vi" "Main VI Log Ref"() -> (w134:refnum<vi>)
            n75 = global read "(Var)System Variables.vi" "IC I2C ID"() -> (w135:u8)
            n76 = call-poly "(SubVI)I2C.vi"("Log Ref"=w134, "error in (no error)"=w110, "Size to Read"=u16 14, "Start Address"=u8 11, "ID"=w135) -> ("error out"=w133:errorcluster, "Read Data"=w130:u8[])  [unwired: 4 in, 1 out]
            n77 = Delete From Array(array=w130, index=0 ("인덱스")) -> (deleted portion=w128:u8, array with subset deleted=w125:u8[])  [unwired: 1 in]
            n78 = Delete From Array(array=w125) -> (deleted portion=w121:u8, array with subset deleted=w123:u8[])  [unwired: 2 in]
            n79 = And(x=w121, y=u8 15) -> (x .and. y?=w120:u8)
            n80 = And(x=w128, y=u8 3) -> (x .and. y?=w127:u8)
            n81 = Delete From Array(array=w123, length=4 ("길이")) -> (deleted portion=w119:u8[], array with subset deleted=w118:u8[])  [unwired: 1 in]
            n82 = local write "Mem Set_Main Seq Loop"(w120) -> ()
            n83 = local write "Mem Set_Gain"(w127) -> ()
            n84 = for {
              tunnel: w118 -> [w147] mode=indexing
              tunnel: [w141] -> w117 mode=indexing
              n85 = Number To Boolean Array(number=w147) -> (Boolean array=w146:bool[])
              n86 = Split 1D Array(array=w146, index=7 ("인덱스")) -> (first subarray=w144:bool[], second subarray=w143:bool[])
              n87 = Boolean Array To Number ("불리언 배열을 숫자로")(Boolean array=w144) -> (number=w142:u8)
              n88 = Boolean Array To Number ("불리언 배열을 숫자로")(Boolean array=w143) -> (number=w140:u8)
              n89 = Bundle(w140, w142) -> (w141:cluster{u8, u8})  [unwired: 1 in]
            }
            n90 = for {
              tunnel: w119 -> [w155] mode=indexing
              tunnel: [w148] -> w116 mode=concatenating
              n91 = Number To Boolean Array(number=w155) -> (Boolean array=w154:bool[])
              n92 = Split 1D Array(array=w154, index=4 ("인덱스")) -> (first subarray=w152:bool[], second subarray=w151:bool[])
              n93 = Boolean Array To Number ("불리언 배열을 숫자로")(Boolean array=w152) -> (number=w150:u8)
              n94 = Boolean Array To Number ("불리언 배열을 숫자로")(Boolean array=w151) -> (number=w149:u8)
              n95 = Build Array(w150, w149) -> (w148:u8[])
            }
            n96 = Array To Cluster(array=w117) -> (cluster=w114:T10)
            n97 = Array To Cluster(array=w116) -> (cluster=w115:T11)
            n98 = property on="Mem Set_Wave Seq" class="Clust (엄격한)"("Value"=w114) -> ("Controls[]"=w113:refnum<vi>[])  [unwired: 2 in, 2 out]
            n99 = control-ref of="Wave Seq. 0"() -> (w112:refnum<vi>)
            n100 = control-ref of="Mem Set_Wave Seq Loop"() -> (w111:refnum<vi>)
            n101 = local write "Mem Set_Wave Seq Loop"(w115) -> ()
            n102 = for {
              tunnel: w113 -> [w138] mode=indexing
              tunnel: w112 -> [w137]
              tunnel: w111 -> [w136]
              n103 = To More Specific Class(target class=w137, reference=w138) -> (specific class reference=w139:refnum<vi>)  [unwired: 1 in, 1 out]
              n104 = call "(DW7912)Update Wave Seq Value Ring.vi"("Wave Seq Loop Ref In"=w136, "Wave Seq Ref In"=w139) -> ()  [unwired: 8 in, 2 out]
            }
          }
          frame "Trig/Interrupt Mode Set" {
            n105 = global read "(Var)System Variables.vi" "Main VI Log Ref"() -> (w169:refnum<vi>)
            n106 = global read "(Var)System Variables.vi" "IC I2C ID"() -> (w170:u8)
            n107 = call-poly "(SubVI)I2C.vi"("Log Ref"=w169, "error in (no error)"=w171, "Address to Read"=T8[] [{"Address"=3, "Delay(ms)"=0}, {"Address"=25, "Delay(ms)"=0}, {"Address"=26, "Delay(ms)"=0}], "ID"=w170) -> ("error out"=w168:errorcluster, "Read Data"=w166:u8[])  [unwired: 5 in, 1 out]
            n108 = Index Array(array=w166) -> (element #1=w165:u8, element #2=w161:u8, element #3=w158:u8)  [unwired: 3 in]
            n109 = Number To Boolean Array(number=w165) -> (Boolean array=w164:bool[])
            n110 = And(x=w161, y=u8 127) -> (x .and. y?=w157:u8)
            n111 = And(x=w158, y=u8 127) -> (x .and. y?=w156:u8)
            n112 = Index Array(array=w164, index=5 ("인덱스")) -> (element=w162:bool)
            n113 = local write "Trig_Mode"(w162) -> ()
            n114 = local write "Trig_R Wave"(w157) -> ()
            n115 = local write "Trig_F Wave"(w156) -> ()
          }
        }
        n116 = call "(SubVI)I2C_Log_Append LF.vi"("Log Ref"=w58, "error in (no error)"=w63) -> ("error out"=w59:errorcluster)  [unwired: 9 in]
        n117 = case shown="에러 .." w59 {
          frame No Error {
          }
          frame Error {
            n118 = control-ref of="Com_Read"() -> (w174:refnum<vi>)
            n119 = control-ref of="Mem Set_Read"() -> (w173:refnum<vi>)
            n120 = control-ref of="Trig_Read"() -> (w172:refnum<vi>)
            n121 = Build Array(w174, w173, w172) -> (w175:refnum<vi>[])
            n122 = Flush Event Queue(2:w175) -> ()  [unwired: 5 in, 3 out]
          }
        }
      }
      event "Com_Mode", "Trig_Mode": Value Change {
        n123 = event-data() -> ()  [unwired: 1 in, 6 out]
        n124 = Boolean To (0,1)(Boolean="Trig_Mode") -> (0, 1=w179:i16)
        n125 = case shown="\"MEM Mode\"" "Com_Mode" {
          tunnel: [w189 T5."Enabled" ("비활성화")] -> w177
          tunnel: [w189 w192] -> w176
          frame "RTP Mode", Default {
            w189 = T5."Disabled and Grayed Out" ("비활성화")
          }
          frame "MEM Mode" {
            n126 = local read "Com_Bst_VD Clamp Reg"() -> (w191:u8)
            n127 = Not Equal To 0?(x=w191) -> (x != 0?=w190:bool)
            n128 = Select(t=T5."Enabled" ("비활성화"), s=w190, f=T5."Disabled and Grayed Out") -> (s? t:f=w192:T5)
          }
        }
        n129 = To Unsigned Byte Integer(number="Com_Mode") -> (unsigned 8bit integer=w182:u8)
        n130 = To Unsigned Byte Integer(number=w179) -> (unsigned 8bit integer=w181:u8)
        n131 = Logical Shift(y=i16 5, x=w181) -> (x << y=w184:u8)
        n132 = global read "(Var)System Variables.vi" "Main VI Log Ref"() -> (w187:refnum<vi>)
        n133 = Or(x=w182, y=w184) -> (x .or. y?=w183:u8)
        n134 = global read "(Var)System Variables.vi" "IC I2C ID"() -> (w188:u8)
        n135 = call-poly "(SubVI)I2C.vi"("Log Ref"=w187, "Data to Write"=w183, "Address"=u8 3, "ID"=w188) -> ()  [unwired: 6 in, 2 out]
        n136 = property on="Com_Bst_VD Clamp Reg" class="Ring (엄격한)"("DisabledEnum"=w177) -> ()  [unwired: 2 in, 2 out]
        n137 = property on="Com_Bst_Wait" class="Ring (엄격한)"("DisabledEnum"=w176) -> ()  [unwired: 2 in, 2 out]
      }
      event "Com_PWM Freq", "Com_Bst_VD Clamp Reg": Value Change {
        # "Waveform Editor에서도 변경되도록 함"
        n138 = event-data() -> ()  [unwired: 1 in, 6 out]
        n139 = Not Equal To 0?(x="Com_Bst_VD Clamp Reg") -> (x != 0?=w197:bool)
        n140 = call "(SubVI)Waveform Editor_Update Sampling Rate Value.vi"("Action"=(Ctrl)Waveform_Editor_Update_Sampling_Rate_Value."Update", "Value"="Com_PWM Freq") -> ()  [unwired: 9 in, 1 out]
        n141 = Logical Shift(y=i16 2, x="Com_Bst_VD Clamp Reg") -> (x << y=w204:u8)
        n142 = global read "(Var)System Variables.vi" "Main VI Log Ref"() -> (w207:refnum<vi>)
        n143 = Or(x="Com_PWM Freq", y=w204) -> (x .or. y?=w203:u8)
        n144 = global read "(Var)System Variables.vi" "IC I2C ID"() -> (w208:u8)
        n145 = Select(t=T5."Enabled" ("비활성화"), s=w197, f=T5."Disabled and Grayed Out") -> (s? t:f=w200:T5)
        n146 = call-poly "(SubVI)I2C.vi"("Log Ref"=w207, "Data to Write"=w203, "Address"=u8 4, "ID"=w208) -> ()  [unwired: 6 in, 2 out]
        n147 = property on="Com_Bst_Wait" class="Ring (엄격한)"("DisabledEnum"=w200) -> ()  [unwired: 2 in, 2 out]
      }
      event "Com_Bst_Mode", "Com_Bst_Wait": Value Change {
        n148 = event-data() -> ()  [unwired: 1 in, 6 out]
        n149 = Logical Shift(y=i16 4, x="Com_Bst_Wait") -> (x << y=w212:u8)
        n150 = global read "(Var)System Variables.vi" "Main VI Log Ref"() -> (w215:refnum<vi>)
        n151 = Or(x="Com_Bst_Mode", y=w212) -> (x .or. y?=w211:u8)
        n152 = global read "(Var)System Variables.vi" "IC I2C ID"() -> (w216:u8)
        n153 = call-poly "(SubVI)I2C.vi"("Log Ref"=w215, "Data to Write"=w211, "Address"=u8 6, "ID"=w216) -> ()  [unwired: 6 in, 2 out]
      }
      event "Com_Bst_VD Clamp": Value Change {
        n154 = event-data() -> ()  [unwired: 1 in, 6 out]
        n155 = global read "(Var)System Variables.vi" "Main VI Log Ref"() -> (w219:refnum<vi>)
        n156 = global read "(Var)System Variables.vi" "IC I2C ID"() -> (w220:u8)
        n157 = call-poly "(SubVI)I2C.vi"("Log Ref"=w219, "Data to Write"="Com_Bst_VD Clamp", "Address"=u8 8, "ID"=w220) -> ()  [unwired: 6 in, 2 out]
      }
      event "Com_Bst_Limit", "Com_Bst_Offset": Value Change {
        n158 = event-data() -> ()  [unwired: 1 in, 6 out]
        n159 = Logical Shift(y=i16 5, x="Com_Bst_Limit") -> (x << y=w224:u8)
        n160 = global read "(Var)System Variables.vi" "Main VI Log Ref"() -> (w227:refnum<vi>)
        n161 = Or(x="Com_Bst_Offset", y=w224) -> (x .or. y?=w223:u8)
        n162 = global read "(Var)System Variables.vi" "IC I2C ID"() -> (w228:u8)
        n163 = call-poly "(SubVI)I2C.vi"("Log Ref"=w227, "Data to Write"=w223, "Address"=u8 35, "ID"=w228) -> ()  [unwired: 6 in, 2 out]
      }
      event Value Change {
        # "Wave Seq. 0 주소\n원소의 인덱스에 따라 주소를 증가"
        n164 = event-data() -> ("CtlRef"=w241:refnum<vi>)  [unwired: 1 in, 5 out]
        n165 = property class="Clust (엄격한)"(reference=w241) -> (reference out=w230:refnum<vi>, "Value"=w229:T2)  [unwired: 1 in, 1 out]
        n166 = control-ref of="Mem Set_Wave Seq Loop"() -> (w231:refnum<vi>)
        n167 = Unbundle(w229) -> ("Mode"=w233:u8, "Seq/Delay"=w238:u8)
        n168 = call "(DW7912)Update Wave Seq Value Ring.vi"("Wave Seq Loop Ref In"=w231, "Wave Seq Ref In"=w230) -> ("index"=w232:u8)  [unwired: 8 in, 1 out]
        n169 = Logical Shift(y=i16 7, x=w233) -> (x << y=w239:u8)
        n170 = Or(x=w239, y=w238) -> (x .or. y?=w237:u8)
        n171 = Add(x=w232, y=u8 12) -> (x+y=w236:u8)
        n172 = global read "(Var)System Variables.vi" "Main VI Log Ref"() -> (w234:refnum<vi>)
        n173 = global read "(Var)System Variables.vi" "IC I2C ID"() -> (w235:u8)
        n174 = call-poly "(SubVI)I2C.vi"("Log Ref"=w234, "Data to Write"=w237, "Address"=w236, "ID"=w235) -> ()  [unwired: 6 in, 2 out]
      }
      event Value Change {
        w247 = refnum<vi> refnum  # 클러스터
        # "FAE3팀에서 Wave Seq.의 Mode 변경 시 \nMem.No의 값을 0으로 변경하도록 요청"
        n175 = event-data() -> ("CtlRef"=w250:refnum<vi>)  [unwired: 1 in, 5 out]
        n176 = property class="Ring (엄격한)"(reference=w250) -> ("Owner"=w249:refnum<vi>)  [unwired: 1 in, 2 out]
        n177 = To More Specific Class(target class=w247, reference=w249) -> (specific class reference=w248:refnum<vi>)  [unwired: 1 in, 1 out]
        n178 = property class="Clust"(reference=w248) -> ("Controls[]"=w246:refnum<vi>[])  [unwired: 1 in, 2 out]
        n179 = Index Array(array=w246, index=1 ("인덱스")) -> (element=w244:refnum<vi>)
        n180 = property class="Ctl"(reference=w244, "Value"=u8 0) -> ()  [unwired: 1 in, 2 out]
      }
      event "Mem Set_Wave Seq Loop.Loop 0", "Mem Set_Wave Seq Loop.Loop 1", "Mem Set_Wave Seq Loop.Loop 2", "Mem Set_Wave Seq Loop.Loop 3", "Mem Set_Wave Seq Loop.Loop 4", "Mem Set_Wave Seq Loop.Loop 5", "Mem Set_Wave Seq Loop.Loop 6", "Mem Set_Wave Seq Loop.Loop 7": Value Change {
        # "Wave Seq Loop의 경우 2개가 1바이트"
        n181 = event-data() -> ("CtlRef"=w262:refnum<vi>)  [unwired: 1 in, 5 out]
        n182 = property on="Mem Set_Wave Seq Loop" class="Clust (엄격한)"() -> ("Controls[]"=w267:refnum<vi>[])  [unwired: 2 in, 2 out]
        n183 = call "Search Unsorted 1D Array.vim"("element"=w262, "unsorted 1D array"=w267) -> ("index of element"=w266:i32)  [unwired: 9 in]
        n184 = Cluster To Array(cluster="Mem Set_Wave Seq Loop") -> (array=w259:u8[])
        n185 = To Unsigned Byte Integer(number=w266) -> (unsigned 8bit integer=w268:u8)
        n186 = Quotient & Remainder(x=w268, y=u8 2) -> (floor(x/y)=w258:u8)  [unwired: 1 out]
        n187 = Multiply(x=w258, y=u8 2) -> (x*y=w252:u8)
        n188 = Add(x=w258, y=u8 20) -> (x+y=w265:u8)
        n189 = Index Array(array=w259, index #1=w252) -> (element #1=w255:u8, element #2=w257:u8)  [unwired: 1 in]
        n190 = global read "(Var)System Variables.vi" "Main VI Log Ref"() -> (w263:refnum<vi>)
        n191 = global read "(Var)System Variables.vi" "IC I2C ID"() -> (w264:u8)
        n192 = Logical Shift(y=i16 4, x=w257) -> (x << y=w254:u8)
        n193 = Or(x=w255, y=w254) -> (x .or. y?=w253:u8)
        n194 = call-poly "(SubVI)I2C.vi"("Log Ref"=w263, "Data to Write"=w253, "Address"=w265, "ID"=w264) -> ()  [unwired: 6 in, 2 out]
      }
      event "Mem Set_Gain": Value Change {
        n195 = event-data() -> ()  [unwired: 1 in, 6 out]
        n196 = global read "(Var)System Variables.vi" "Main VI Log Ref"() -> (w272:refnum<vi>)
        n197 = global read "(Var)System Variables.vi" "IC I2C ID"() -> (w273:u8)
        n198 = call-poly "(SubVI)I2C.vi"("Log Ref"=w272, "Data to Write"="Mem Set_Gain", "Address"=u8 11, "ID"=w273) -> ()  [unwired: 6 in, 2 out]
      }
      event "Mem Set_Main Seq Loop": Value Change {
        n199 = event-data() -> ()  [unwired: 1 in, 6 out]
        n200 = global read "(Var)System Variables.vi" "Main VI Log Ref"() -> (w276:refnum<vi>)
        n201 = global read "(Var)System Variables.vi" "IC I2C ID"() -> (w277:u8)
        n202 = call-poly "(SubVI)I2C.vi"("Log Ref"=w276, "Data to Write"="Mem Set_Main Seq Loop", "Address"=u8 24, "ID"=w277) -> ()  [unwired: 6 in, 2 out]
      }
      event "Mem_Start", "Mem_Stop": Value Change {
        # "Stop 이벤트 시 0\nStart 이벤트 시 1"
        n203 = event-data() -> ()  [unwired: 1 in, 6 out]
        n204 = Boolean To (0,1)(Boolean="Mem_Start") -> (0, 1=w280:i16)
        n205 = To Unsigned Byte Integer(number=w280) -> (unsigned 8bit integer=w279:u8)
        n206 = global read "(Var)System Variables.vi" "Main VI Log Ref"() -> (w282:refnum<vi>)
        n207 = global read "(Var)System Variables.vi" "IC I2C ID"() -> (w283:u8)
        n208 = call-poly "(SubVI)I2C.vi"("Log Ref"=w282, "Data to Write"=w279, "Address"=u8 9, "ID"=w283) -> ()  [unwired: 6 in, 2 out]
      }
      event "Trig_R Wave", "Trig_F Wave": Value Change {
        n209 = event-data() -> ("CtlRef"=w287:refnum<vi>, "NewVal"=w284:u8)  [unwired: 1 in, 4 out]
        n210 = property class="Ring (엄격한)"(reference=w287) -> ("Label.Text"=w286:string)  [unwired: 1 in, 2 out]
        n211 = case shown="\"Trig_R Wave\", 기본" w286 {
          tunnel: [u8 25 u8 26] -> w285
          frame "Trig_R Wave", Default {
          }
          frame "Trig_F Wave" {
          }
        }
        n212 = global read "(Var)System Variables.vi" "Main VI Log Ref"() -> (w288:refnum<vi>)
        n213 = global read "(Var)System Variables.vi" "IC I2C ID"() -> (w289:u8)
        n214 = call-poly "(SubVI)I2C.vi"("Log Ref"=w288, "Data to Write"=w284, "Address"=w285, "ID"=w289) -> ()  [unwired: 6 in, 2 out]
      }
      event Value Change {
        # "Trigger 설정에 따른 그림 생성"
        # "비활성화, 시간 설정 범위 관련 처리"
        n215 = event-data() -> ("CtlRef"=w296:refnum<vi>)  [unwired: 1 in, 5 out]
        n216 = call "(SubVI)Update Trigger Control Cluster.vi"("Trig Ctrl Ref"=w296) -> ("Disable"=w295:T5)  [unwired: 9 in, 1 out]
        n217 = property on="Trig_Gen_Set" class="Bool"("DisabledEnum"=w295) -> ()  [unwired: 2 in, 2 out]
        n218 = call "(SubVI)GPIO Trigger Picture.vi"("num of ch (4)"=2, "Trig Ctrl"="Trig_Gen_Setting") -> ("picture"=→"Trig_Gen_Pict":picture)  [unwired: 9 in]
      }
      event "Trig_Gen_Set": Value Change {
        # "트리거 발생"
        n219 = event-data() -> ()  [unwired: 1 in, 6 out]
        n220 = local read "Trig_Gen_Setting"() -> (w297:T4)
        n221 = call "(SubVI)System Command_Trig GPIO Control.vi"("Trig_Ctrl"=w297) -> ()  [unwired: 10 in, 1 out]
      }
    }
    n222 = global read "(Var)System Variables.vi" "Quit System"() -> (w30:bool)
    n223 = Or(x="Stop", y=w30) -> (x .or. y?=w28:bool)
  }
  n224 = flat-sequence {
    tunnel: w18 -> [_]
    frame #0 {
      # "Trigger 설정 값 저장"
      n225 = control-ref of="Trig_Gen_Setting"() -> (w301:refnum<vi>)
      n226 = Build Array(w301) -> (w300:refnum<vi>[])
      n227 = call "(SubVI)Control Data_Save or Load Control Value.vi"("Common? (f)"=TRUE, "Function"=(Ctrl)Control_Data_Save_or_Load_Control_Data_Function."Save", "Control Ref"=w300) -> ()  [unwired: 8 in, 1 out]
    }
  }
